vi "Acquisition_Order.vi"(1 "Vi Name":string) -> (0 "Acquisition Order":T1)   [LabVIEW 2017]
uses:
  Acquisition_Order.ctl
  Globals/Meas_global.vi
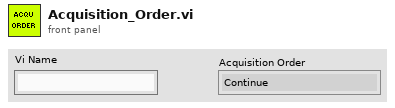
[diagram p1: front panel]
types:
  T1 = typedef "Acquisition_Order.ctl" = enum16{"Continue", "Set Occurrence", "Wait on Occurrence"}
  T2 = typedef "Trigger_Mode.ctl" = enum16{"Free Running", "Start on Trigger", "Trigger Every Block", "Trigger Every Sample"}
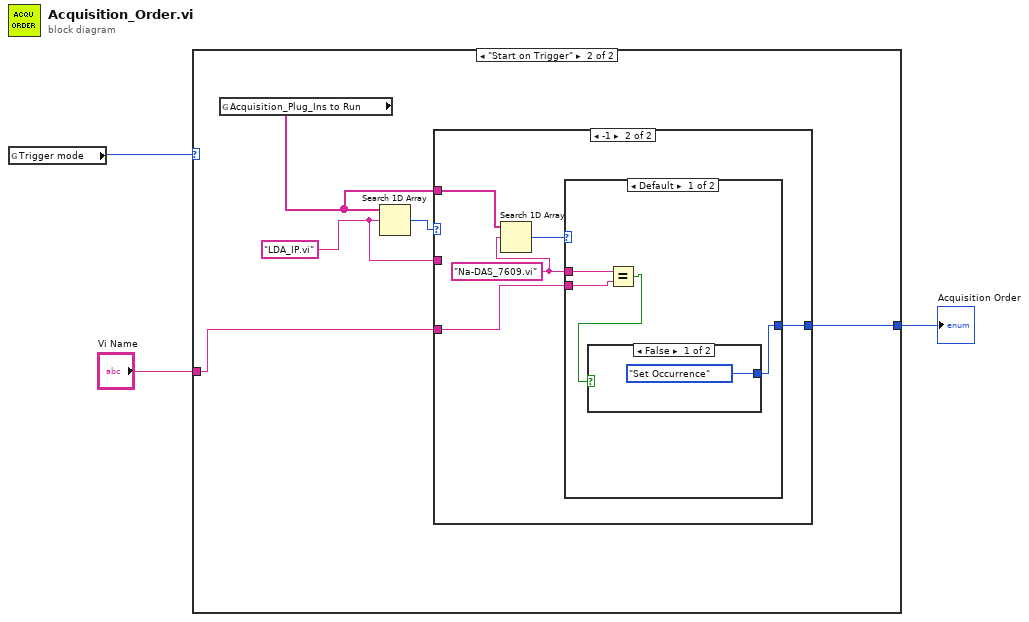
[diagram p0: block diagram]
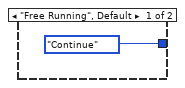
[diagram p2: hidden frame]
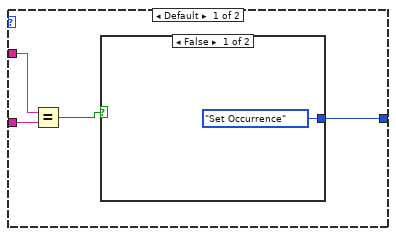
[diagram p3: hidden frame]
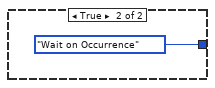
[diagram p4: hidden frame]
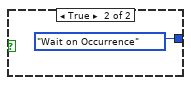
[diagram p5: hidden frame]
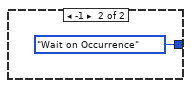
[diagram p6: hidden frame]
diagram:
  n1 = global read "Meas_global.vi" "Trigger mode"() -> (w3:T2)
  n2 = case shown="\"Start on Trigger\"" w3 {
    tunnel: [Acquisition_Order."Continue" ("Acquisition Order") w6] -> w2
    tunnel: "Vi Name" -> [_ w7]
    frame "Free Running", Default {
    }
    frame "Start on Trigger" {
      w8 = "LDA_IP.vi"
      n3 = global read "Meas_global.vi" "Acquisition_Plug_Ins to Run"() -> (w5:string[])
      n4 = Search 1D Array(1D array=w5, element=w8) -> (index of element=w9:i32)  [unwired: 1 in]
      n5 = case shown="-1" w9 {
        tunnel: w8 -> [w13 _]
        tunnel: w7 -> [w12 w17]
        tunnel: [w11 w16] -> w6
        tunnel: w5 -> [_ w20]
        frame Default {
          n6 = Equal?(x=w13, y=w12) -> (x = y?=w10:bool)
          n7 = case shown="False" w10 {
            tunnel: [Acquisition_Order."Set Occurrence" ("Acquisition Order") Acquisition_Order."Wait on Occurrence" ("Acquisition Order")] -> w11
            frame False {
            }
            frame True {
            }
          }
        }
        frame -1 {
          w18 = "Na-DAS_7609.vi"
          n8 = Search 1D Array(1D array=w20, element=w18) -> (index of element=w19:i32)  [unwired: 1 in]
          n9 = case shown="Default" w19 {
            tunnel: w18 -> [w24 _]
            tunnel: w17 -> [w23 _]
            tunnel: [w21 Acquisition_Order."Wait on Occurrence" ("Acquisition Order")] -> w16
            frame Default {
              n10 = Equal?(x=w24, y=w23) -> (x = y?=w22:bool)
              n11 = case shown="False" w22 {
                tunnel: [Acquisition_Order."Set Occurrence" ("Acquisition Order") Acquisition_Order."Wait on Occurrence" ("Acquisition Order")] -> w21
                frame False {
                }
                frame True {
                }
              }
            }
            frame -1 {
            }
          }
        }
      }
    }
  }
  "Acquisition Order" <- w2
